vi "CheckType (SubVI).vi"(10 "Тип/версия устройства":string, 11 "paramUnicornIn in":T1) -> (3 "Connection":bool)   [LabVIEW 2017, in "LV_Unicorn.lvlib"]
uses:
  LV_Unicorn.lvlib
  Control/unicorn_Param.ctl
  Control/unicorn_conn.ctl
  Control/unicorn_JSON.ctl
  Control/unicorn_ParamInt.ctl
  Control/unicorn_Telemetry.ctl
  Control/unicorn_Table.ctl
  Control/unicorn_ParamFloat.ctl
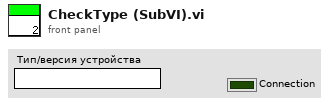
[diagram p1: front panel]
types:
  T1 = typedef "LV_Unicorn.lvlib/unicorn_Param.ctl" = cluster{"conParam":T2, "Param":T3}
  T2 = typedef "LV_Unicorn.lvlib/unicorn_conn.ctl" = cluster{"ReadIntParam":bool, "ReadDescrParam":bool, "ReadFloatParam":bool, "debug":bool, "ReadJSON":bool, "IP_address":string, "N_attempts":i32, "type_con":enum16{"Serial", "TCP"}, "MB_address":i32, "VISA":refnum<visa-resource-name>, "connection ID":refnum<k5>, "nameDevices":string, "timeout":i32, "port":u16, "type_version":string, "baud_rate":u32, "VersionControl":bool, "TCP_conn":bool, "WindowSize":i32}
  T3 = typedef "LV_Unicorn.lvlib/unicorn_JSON.ctl" = cluster{"NumParam":cluster{"NTelem":i32, "NInt":i32, "NFloat":i32, "NTable":i32}, "ParamInt":T4, "Telemetry":T5, "Table":T6, "ParamFloat":T7}
  T4 = typedef "LV_Unicorn.lvlib/unicorn_ParamInt.ctl" = cluster{"ID":string, "Num":i32, "Name":string, "Type":string, "Enum":string, "Desc":string, "Unit":string, "Access":string, "FormatStr":string, "Min":i32, "Max":i32}[]
  T5 = typedef "LV_Unicorn.lvlib/unicorn_Telemetry.ctl" = cluster{"ID":string, "Num":i32, "Name":string, "Desc":string, "Unit":string, "FormatStr":string, "Min":i32, "Max":i32}[]
  T6 = typedef "LV_Unicorn.lvlib/unicorn_Table.ctl" = cluster{"Num":i32, "Access":string, "ColumnCount":i32, "NeedParamPrepare":bool, "Columns":cluster{"Column":i32, "Desc":string, "Name":string}[], "DataType":string, "FormatStr":string, "ID":string, "Name":string, "RowCount":i32, "Rows":cluster{"Desc":string, "ID":string, "Max":i32, "Min":i32, "Name":string, "Row":i32, "Unit":string}[], "Type":string}[]
  T7 = typedef "LV_Unicorn.lvlib/unicorn_ParamFloat.ctl" = cluster{"ID":string, "Num":i32, "Name":string, "Type":string, "Enum":string, "Desc":string, "Unit":string, "Access":string, "FormatStr":string, "Min":sgl, "Max":sgl}[]
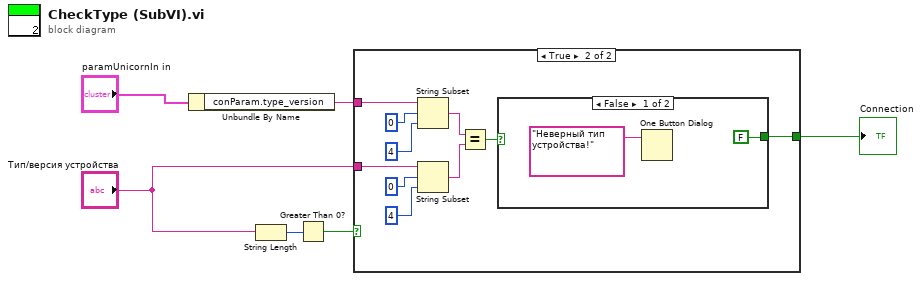
[diagram p0: block diagram]
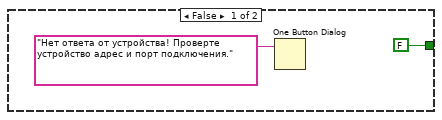
[diagram p2: hidden frame]
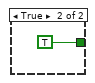
[diagram p3: hidden frame]
diagram:
  n1 = Unbundle By Name("paramUnicornIn in") -> ("conParam.type_version"=w5:string)
  n2 = String Length(string="Тип/версия устройства") -> (length=w1:i32)
  n3 = Greater Than 0?(x=w1) -> (x > 0?=w2:bool)
  n4 = case shown="True" w2 {
    tunnel: "Тип/версия устройства" -> [_ w14]
    tunnel: w5 -> [_ w11]
    tunnel: [FALSE w9] -> w6
    frame False {
      n5 = One Button Dialog(message="Нет ответа от устройства! Проверте устройство адрес и порт подключения.") -> ()  [unwired: 1 in, 1 out]
    }
    frame True {
      n6 = String Subset(string=w11, offset (0)=0, length (rest)=4 ("length (rest)")) -> (substring=w17:string)
      n7 = String Subset(string=w14, offset (0)=0, length (rest)=4 ("length (rest)")) -> (substring=w18:string)
      n8 = Equal?(x=w17, y=w18) -> (x = y?=w10:bool)
      n9 = case shown="False" w10 {
        tunnel: [FALSE TRUE] -> w9
        frame False {
          n10 = One Button Dialog(message="Неверный тип устройства!") -> ()  [unwired: 1 in, 1 out]
        }
        frame True {
        }
      }
    }
  }
  "Connection" <- w6
